vi "Periodic Tasks.vi"(8 "error in":errorcluster) -> ()   [LabVIEW 2013]
doc: "This VI runs in parallel to other tasks. It can contain as many user-defined periodic loops as you need. These can carry out PID or other sorts of timed response."
uses:
  <vilib>/Rock Robotics/WPI/DriverStation/DriverStationLCD/WPI_DriverStationLCDLCDLine.ctl
  <vilib>/Rock Robotics/SystemInterfaces/Utilities/FPGA_UtilitiesLED Source.ctl
  <vilib>/Rock Robotics/SystemInterfaces/Utilities/FPGA_UtilitiesLED State.ctl
  <vilib>/Rock Robotics/WPI/DriverStation/WPI_DriverStationRobotMode2.ctl
  <vilib>/Rock Robotics/WPI/SafetyOutput/WPI_SafetyOutputConfigMenu.ctl
  <vilib>/Rock Robotics/WPI/Solenoid/WPI_SolenoidValue.ctl
  <vilib>/Rock Robotics/WPI/Relay/WPI_RelayValue.ctl
  Begin/Global Refnums.vi
  Begin/Robot Global Data.vi
  <vilib>/Rock Robotics/WPI/Solenoid/WPI_SolenoidSetEnum.vi
  Begin/Global Variables.vi
  <vilib>/Rock Robotics/WPI/Joystick/WPI_JoystickGetSetRefNum.vi
  <vilib>/Rock Robotics/WPI/Compressor/WPI_CompressorGetSetRefNum.vi
panel:
  out "Fire":bool
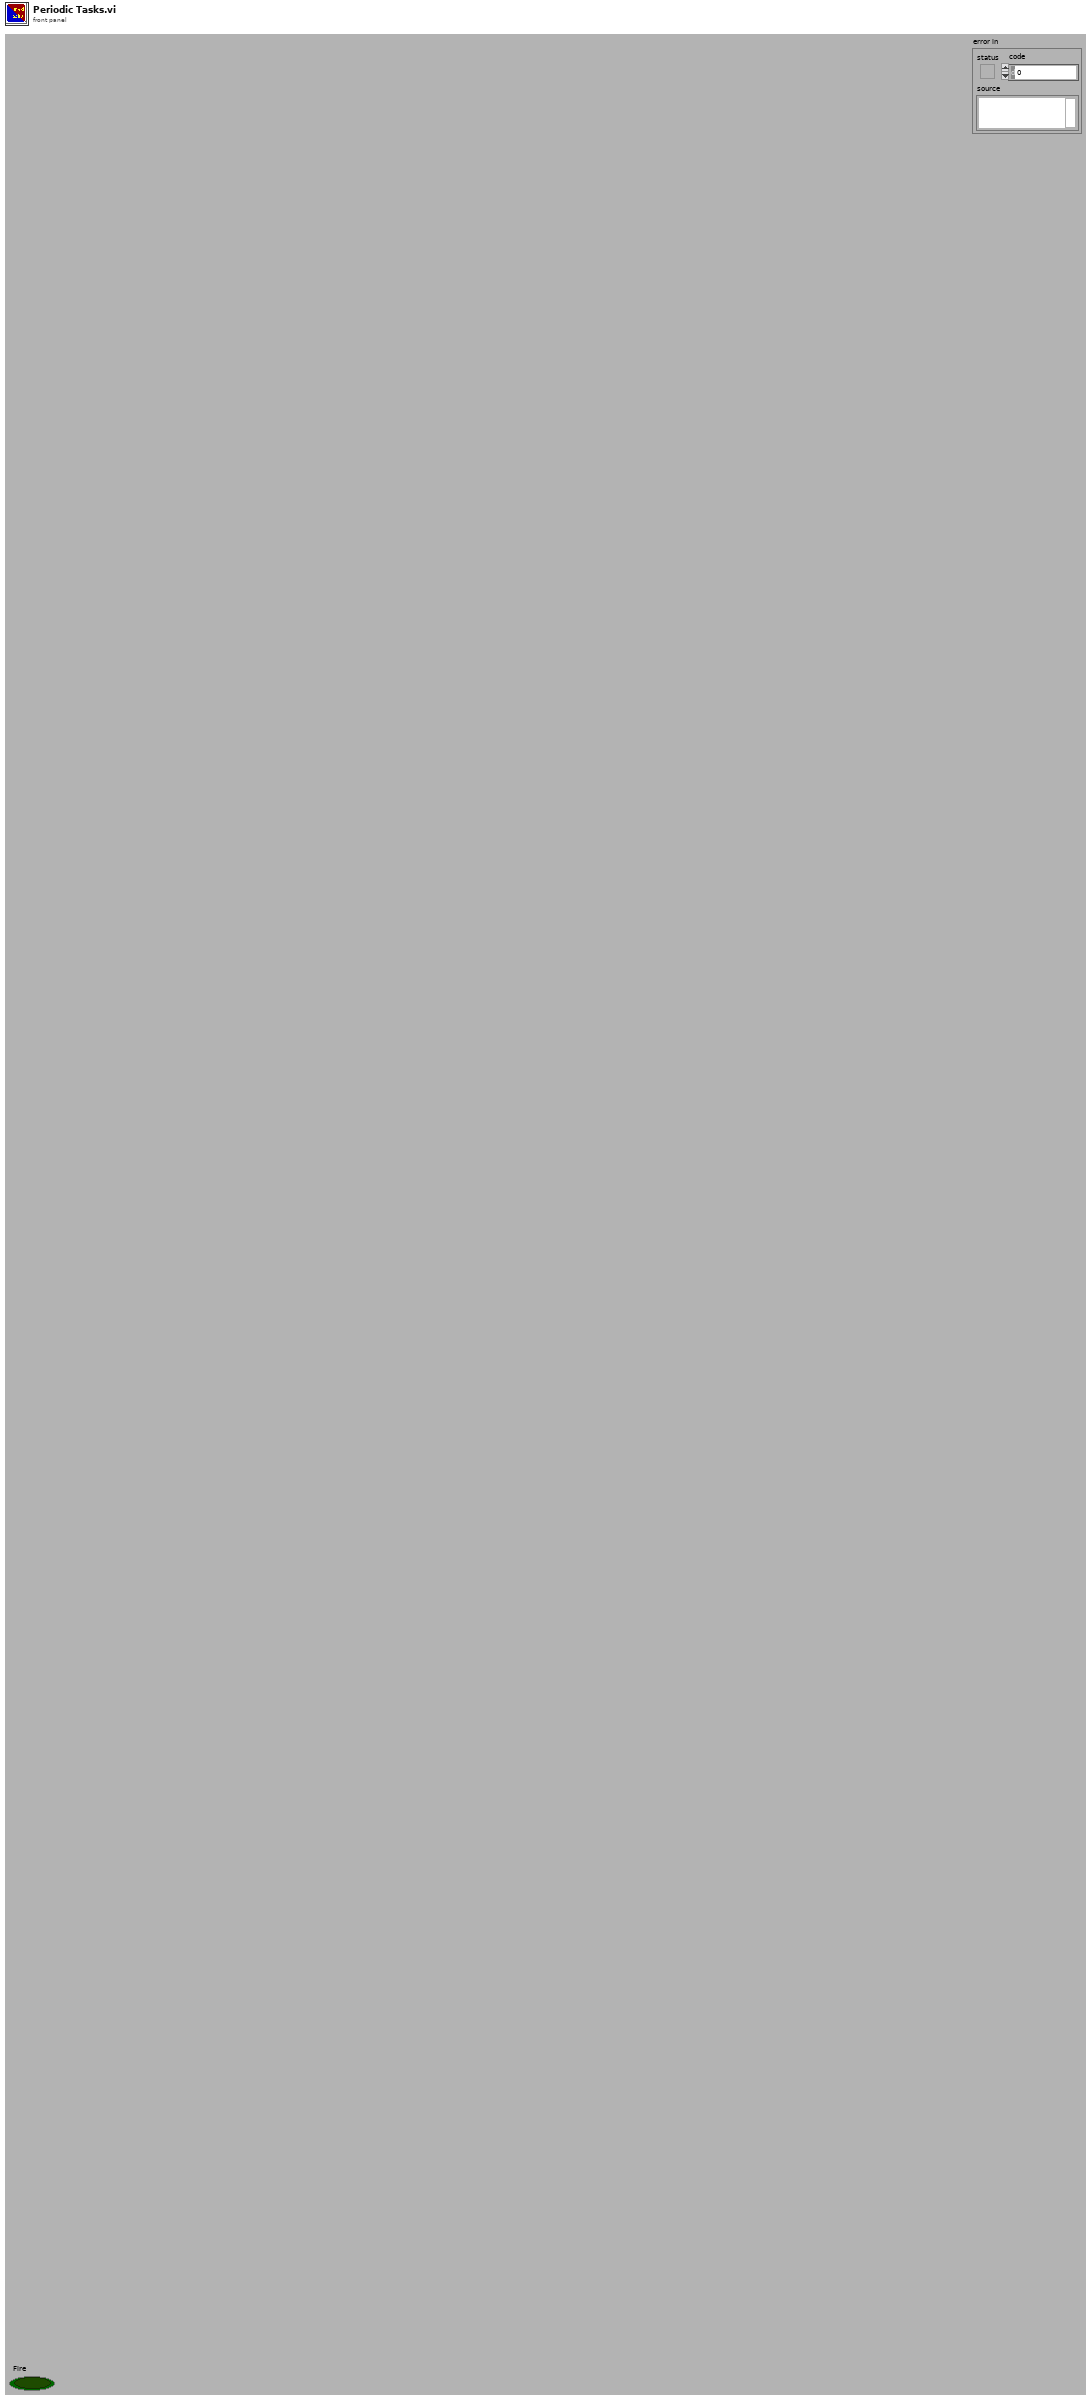
[diagram p1: front panel]
types:
  T1 = typedef "WPI_DriverStationLCDLCDLine.ctl" = enum16{"Main - Line 1", "User - Line 2", "User - Line 3", "User - Line 4", "User - Line 5", "User - Line 6"}
  T2 = typedef "WPI_DriverStationRobotMode2.ctl" = enum16{"Autonomous Disabled", "Autonomous Enabled", "Teleop Disabled", "Teleop Enabled", "Timeout", "Finish", "Test Disabled", "Test Enabled"}
  T3 = typedef "WPI_CompressorDevRef.ctl" = cluster{"DevStatus":errorcluster, "DigitalInputDevRef":T4, "RelayDevRef":T7}
  T4 = typedef "WPI_DigitalInputDevRef.ctl" = cluster{"DevStatus":errorcluster, "DIO Channel":T5, "Digital Module":T6}
  T5 = typedef "FPGA_DIOChannel.ctl" = enum8{"DIO 1", "DIO 2", "DIO 3", "DIO 4", "DIO 5", "DIO 6", "DIO 7", "DIO 8", "DIO 9", "DIO 10", "DIO 11", "DIO 12", "DIO 13", "DIO 14", "Invalid"}
  T6 = typedef "FPGA_TypedefDigitalModule.ctl" = enum16{"Digital Module 1", "Digital Module 2"}
  T7 = typedef "WPI_RelayDevRef.ctl" = cluster{"DevStatus":errorcluster, "Relay Channel":T8, "Digital Module":T6, "Relay Direction":T9}
  T8 = typedef "FPGA_DIORelayChannel.ctl" = enum8{"Relay 1", "Relay 2", "Relay 3", "Relay 4", "Relay 5", "Relay 6", "Relay 7", "Relay 8", "Invalid"}
  T9 = typedef "WPI_RelayDirection.ctl" = enum16{"Both directions", "Forward only", "Reverse only"}
  T10 = typedef "WPI_SolenoidValue.ctl" = enum16{"Off", "On", "Forward", "Reverse"}
  T11 = typedef "WPI_SafetyOutputConfigMenu.ctl" = enum16{"Enable", "Disable"}
  T12 = typedef "WPI_SolenoidDevRef.ctl" = cluster{"DevStatus":errorcluster, "Solenoid Module":T13, "Forward Solenoid Channel":T14, "Reverse Solenoid Channel":T14}
  T13 = typedef "FPGA_TypedefSolenoidModule.ctl" = enum16{"Solenoid Module 1", "Solenoid Module 2"}
  T14 = typedef "WPI_SolenoidChannel.ctl" = enum8{"Solenoid 1", "Solenoid 2", "Solenoid 3", "Solenoid 4", "Solenoid 5", "Solenoid 6", "Solenoid 7", "Solenoid 8", "Invalid"}
  T15 = typedef "WPI_RelayValue.ctl" = enum16{"Off", "On", "Forward", "Reverse"}
  T16 = typedef "WPI_EncoderDevRef.ctl" = cluster{"DevStatus":errorcluster, "EncoderIndex":T17, "CounterIndex":T18, "DistancePerCount":dbl, "Decoding Type":T19}
  T17 = typedef "FPGA_EncoderIdx.ctl" = enum8{"Enc 0", "Enc 1", "Enc 2", "Enc 3", "Invalid"}
  T18 = typedef "FPGA_CounterCtrSystemIndex.ctl" = enum8{"Ctr 0", "Ctr 1", "Ctr 2", "Ctr 3", "Ctr 4", "Ctr 5", "Ctr 6", "Ctr 7", "Invalid"}
  T19 = typedef "WPI_EncoderType.ctl" = enum16{"1x", "2x", "4x"}
  T20 = typedef "WPI_JoystickDevRef.ctl" = cluster{"Device":T21}
  T21 = typedef "WPI_JoystickDeviceEnum.ctl" = enum16{"USB 1", "USB 2", "USB 3", "USB 4", "Kinect 1", "Kinect 2"}
  T22 = typedef "WPI_JoystickButtonState.ctl" = cluster{"Button 1":bool, "Button 2":bool, "Button 3":bool, "Button 4":bool, "Button 5":bool, "Button 6":bool, "Button 7":bool, "Button 8":bool, "Button 9":bool, "Button 10":bool, "Button 11":bool, "Button 12":bool}
  T23 = typedef "WPI_MotorControlDeviceRef.ctl" = cluster{"DeviceStatus":errorcluster, "Type":enum16{"PWM", "CAN"}, "PWM":cluster{"Digital Module":T6, "PWM Channel":T24, "DeadBand":T25}, "CAN":cluster{"Device Number":u8, "Control Mode":T26, "Semaphore":T27, "Max Vout":dbl}, "Invert":bool, "TransformRef":T28, "InvTransformRef":T28}
  T24 = typedef "FPGA_DIOPWMChannel.ctl" = enum8{"PWM 1", "PWM 2", "PWM 3", "PWM 4", "PWM 5", "PWM 6", "PWM 7", "PWM 8", "PWM 9", "PWM 10", "Invalid"}
  T25 = typedef "WPI_PWMDeadband.ctl" = cluster{"Name":string, "maxPositivePwm":i32, "minPositivePwm":i32, "centerPwm":i32, "maxNegativePwm":i32, "minNegativePwm":i32, "angularRange":u16}
  T26 = typedef "WPI_CANJaguar_ControlMode.ctl" = enum8{"Percent VBus", "Current", "Speed", "Position", "Voltage"}
  T27 = typedef "Semaphore RefNum" = refnum<k1>
  T28 = typedef "WPI_PWMTransform_ConPane.ctl" = refnum<vi>
  T29 = typedef "FPGA_UtilitiesLED State.ctl" = enum16{"Off", "On", "Toggle"}
  T30 = typedef "FPGA_UtilitiesLED Source.ctl" = enum16{"User LED", "FPGA LED"}
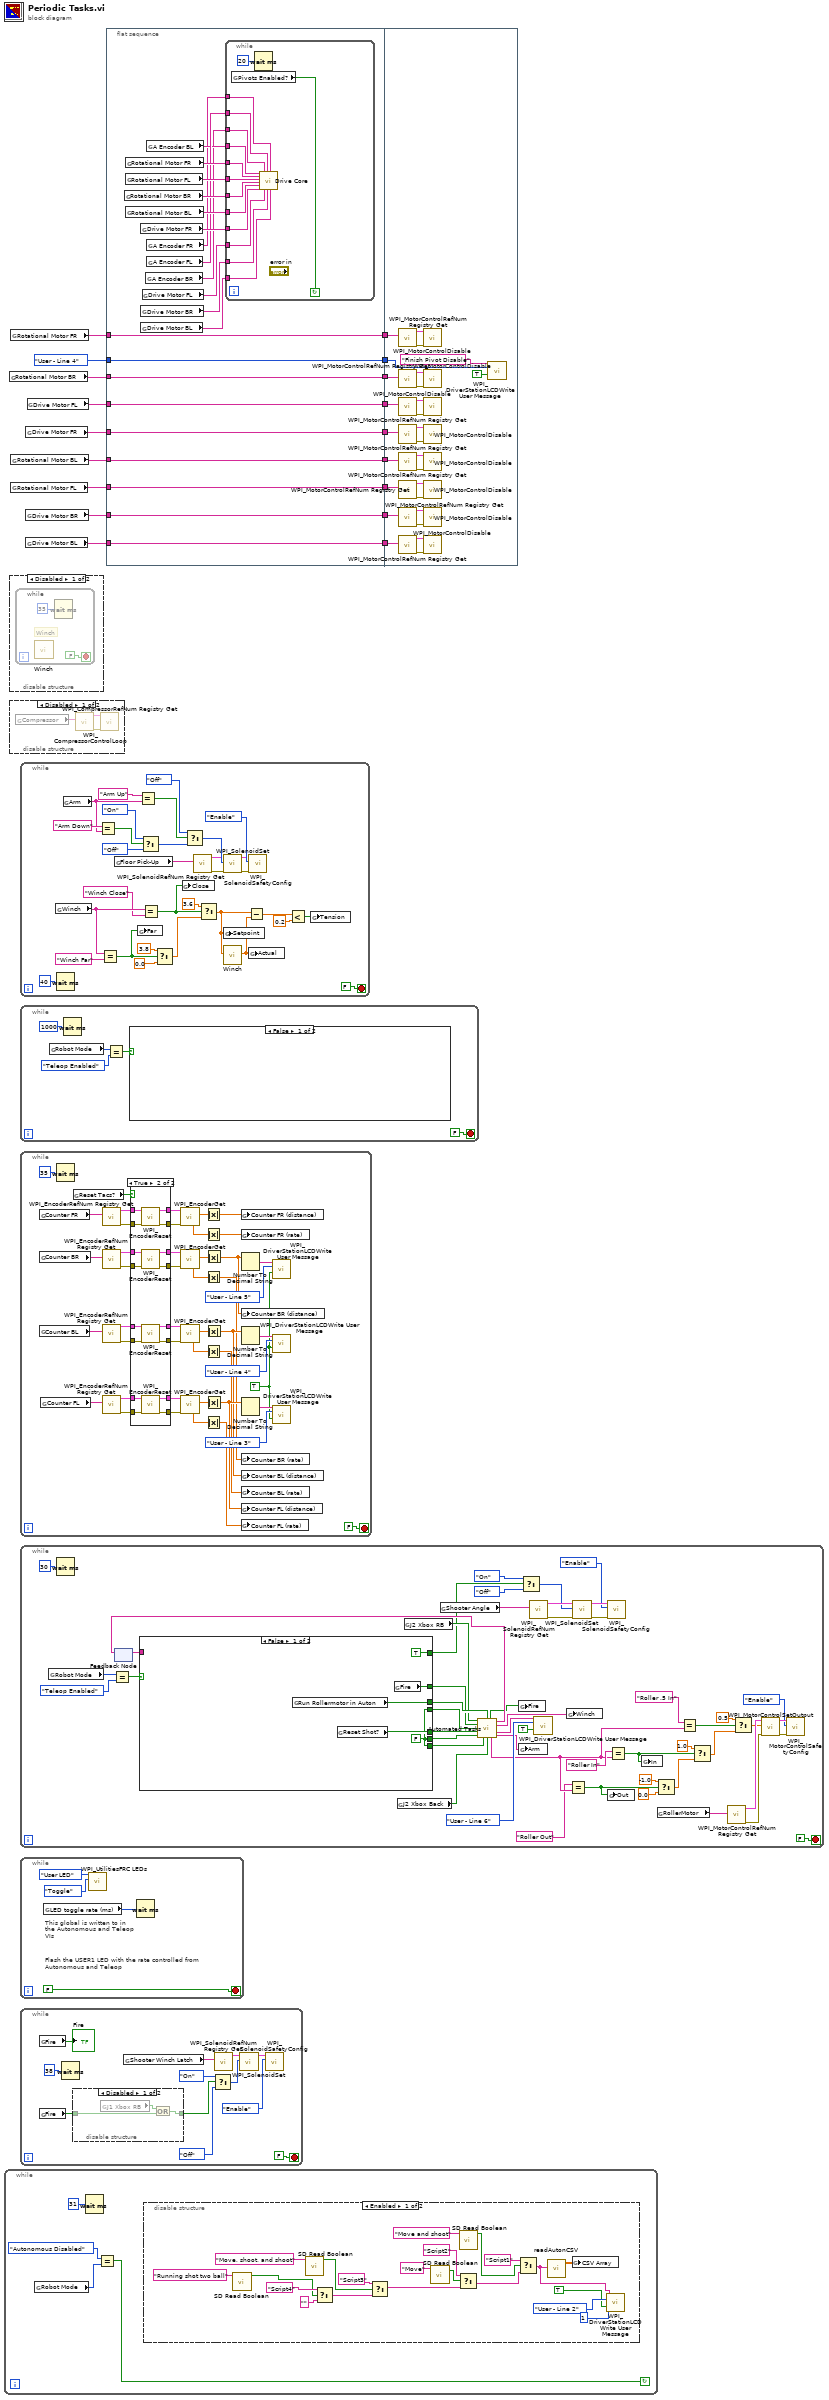
[diagram p0: block diagram]
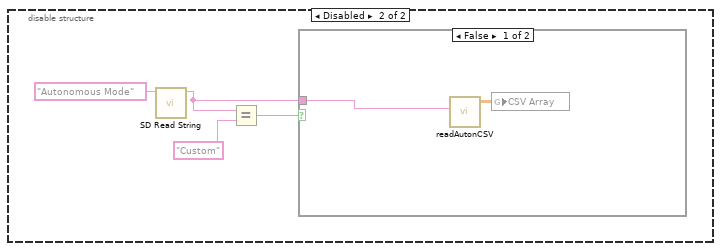
[diagram p2: hidden frame]
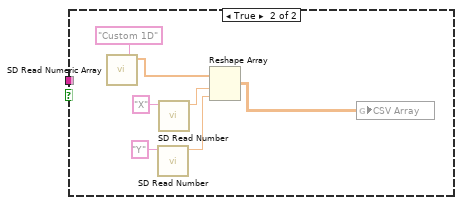
[diagram p3: hidden frame]
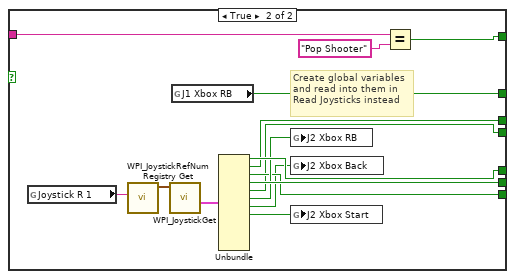
[diagram p6: hidden frame]
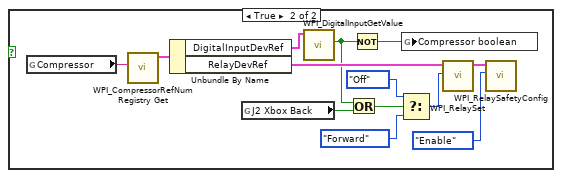
[diagram p8: hidden frame]
diagram:
  n1 = while {
    stop <- w19 continue-if-true
    n2 = global read "Robot Global Data.vi" "Robot Mode"() -> (w21:T2)
    n3 = Wait (ms)(milliseconds to wait=u32 31) -> ()  [unwired: 1 out]
    n4 = Equal?(x=WPI_DriverStationRobotMode2."Autonomous Disabled" ("y"), y=w21) -> (x = y?=w19:bool)
    n5 = disable-structure shown="Enabled" {
      frame Enabled {
        n6 = call <vilib>:"SD Read Boolean.vi"("Name"="Running shot two ball") -> ("Boolean"=w31:bool)  [unwired: 8 in, 2 out]
        n7 = call <vilib>:"SD Read Boolean.vi"("Name"="Move, shoot, and shoot") -> ("Boolean"=w36:bool)  [unwired: 8 in, 2 out]
        n8 = Select(t="Script4" ("Name"), s=w31, f="" ("Name")) -> (s? t:f=w29:string)
        n9 = Select(t="Script3" ("Name"), s=w36, f=w29) -> (s? t:f=w34:string)
        n10 = call <vilib>:"SD Read Boolean.vi"("Name"="Move") -> ("Boolean"=w41:bool)  [unwired: 8 in, 2 out]
        n11 = call <vilib>:"SD Read Boolean.vi"("Name"="Move and shoot") -> ("Boolean"=w39:bool)  [unwired: 8 in, 2 out]
        n12 = Select(t="Script2" ("Name"), s=w41, f=w34) -> (s? t:f=w40:string)
        n13 = Select(t="Script1" ("Name"), s=w39, f=w40) -> (s? t:f=w24:string)
        n14 = call "readAutonCSV.vi"("AutonFile"=w24) -> ("AutonArray"=w27:dbl[][])  [unwired: 7 in]
        n15 = global write "Global Refnums.vi" "CSV Array"(w27) -> ()
        n16 = call <vilib>:"WPI_DriverStationLCDWrite User Message.vi"("line text"=w24, "line"=WPI_DriverStationLCDLCDLine."User - Line 2", "starting column"=i8 1, "clear line before write (T)"=TRUE) -> ()  [unwired: 11 in, 1 out]
      }
      frame Disabled {
        n17 = call <vilib>:"SD Read String.vi"("Name"="Autonomous Mode") -> ("String"=w44:string)  [unwired: 8 in, 2 out]
        n18 = Equal?(x=w44, y="Custom") -> (x = y?=w45:bool)
        n19 = case shown="False" w45 {
          tunnel: w44 -> [w48 _]
          frame False {
            n20 = call "readAutonCSV.vi"("AutonFile"=w48) -> ("AutonArray"=w49:dbl[][])  [unwired: 7 in]
            n21 = global write "Global Refnums.vi" "CSV Array"(w49) -> ()
          }
          frame True {
            n22 = call <vilib>:"SD Read Numeric Array.vi"("Name"="Custom 1D") -> ("Numeric Array"=w55:dbl[])  [unwired: 8 in, 2 out]
            n23 = call <vilib>:"SD Read Number.vi"("Name"="Y") -> ("Numeric"=w51:dbl)  [unwired: 8 in, 2 out]
            n24 = call <vilib>:"SD Read Number.vi"("Name"="X") -> ("Numeric"=w54:dbl)  [unwired: 8 in, 2 out]
            n25 = Reshape Array(w55, w54, w51) -> (w50:dbl[][])
            n26 = global write "Global Refnums.vi" "CSV Array"(w50) -> ()
          }
        }
      }
    }
  }
  n27 = global read "Global Refnums.vi" "Rotational Motor BR"() -> (w16:string)
  n28 = disable-structure shown="Disabled" {
    frame Disabled {
      n29 = while {
        stop <- FALSE stop-if-true
        # "Winch"
        n30 = call "Winch.vi"() -> ()  [unwired: 11 in, 1 out]
        n31 = Wait (ms)(milliseconds to wait=u32 35) -> ()  [unwired: 1 out]
      }
    }
    frame Enabled {
    }
  }
  n32 = disable-structure shown="Disabled" {
    frame Disabled {
      n33 = global read "Global Refnums.vi" "Compressor"() -> (w61:string)
      n34 = call <vilib>:"WPI_CompressorRefNum Registry Get.vi"("refnum name"=w61) -> ("error out"=w60:errorcluster, "CompressorDevRef"=w59:T3)  [unwired: 9 in]
      n35 = call <vilib>:"WPI_CompressorControlLoop.vi"("error in (no error)"=w60, "CompressorDevRef"=w59) -> ()  [unwired: 10 in]
    }
    frame Enabled {
    }
  }
  n36 = global read "Global Refnums.vi" "Rotational Motor FR"() -> (w18:string)
  n37 = global read "Global Refnums.vi" "Rotational Motor BL"() -> (w15:string)
  n38 = global read "Global Refnums.vi" "Rotational Motor FL"() -> (w17:string)
  n39 = while {
    stop <- FALSE stop-if-true
    n40 = global read "Global Refnums.vi" "Winch"() -> (w93:string)
    n41 = Wait (ms)(milliseconds to wait=u32 40) -> ()  [unwired: 1 out]
    n42 = global read "Global Refnums.vi" "Arm"() -> (w67:string)
    n43 = Equal?(x="Arm Down", y=w67) -> (x = y?=w71:bool)
    n44 = Equal?(x=w93, y="Winch Far") -> (x = y?=w64:bool)
    n45 = global read "Global Refnums.vi" "Floor Pick-Up"() -> (w82:string)
    n46 = global write "Global Refnums.vi" "Far"(w64) -> ()
    n47 = Equal?(x="Arm Up", y=w67) -> (x = y?=w84:bool)
    n48 = Select(t=WPI_SolenoidValue."On" ("Value"), s=w71, f=WPI_SolenoidValue."Off" ("Value")) -> (s? t:f=w70:T10)
    n49 = Equal?(x=w93, y="Winch Close") -> (x = y?=w63:bool)
    n50 = Select(t=3.8, s=w64, f=0.0) -> (s? t:f=w90:dbl)
    n51 = global write "Global Refnums.vi" "Close"(w63) -> ()
    n52 = Select(t=WPI_SolenoidValue."Off" ("Value"), s=w84, f=w70) -> (s? t:f=w86:T10)
    n53 = call <vilib>:"WPI_SolenoidRefNum Registry Get.vi"("refnum name"=w82) -> ("error out"=w77:errorcluster, "SolenoidDevRef"=w78:T12)  [unwired: 9 in]
    n54 = Select(t=3.6, s=w63, f=w90) -> (s? t:f=w62:dbl)
    n55 = call-poly <vilib>:"WPI_SolenoidSet.vi"("error in (no error)"=w77, "Value"=w86, "SolenoidDevRef"=w78) -> ("error out"=w80:errorcluster, "SolenoidDevRef"=w79:T12)  [unwired: 7 in]
    n56 = global write "Global Refnums.vi" "Setpoint"(w62) -> ()
    n57 = call "Winch.vi"("setpoint"=w62) -> ("Actual"=w65:dbl)  [unwired: 10 in]
    n58 = Subtract(x=w62, y=w65) -> (x-y=w74:dbl)
    n59 = call <vilib>:"WPI_SolenoidSafetyConfig.vi"("error in (no error)"=w80, "mode"=WPI_SafetyOutputConfigMenu."Enable", "SolenoidDevRef"=w79) -> ()  [unwired: 7 in, 2 out]
    n60 = global write "Global Refnums.vi" "Actual"(w65) -> ()
    n61 = Less?(x=w74, y=0.2) -> (x < y?=w66:bool)
    n62 = global write "Global Refnums.vi" "Tension"(w66) -> ()
  }
  n63 = while {
    stop <- FALSE stop-if-true
    n64 = global read "Robot Global Data.vi" "Robot Mode"() -> (w96:T2)
    n65 = Wait (ms)(milliseconds to wait=1000) -> ()  [unwired: 1 out]
    n66 = Equal?(x=w96, y=WPI_DriverStationRobotMode2."Teleop Enabled") -> (x = y?=w94:bool)
    n67 = case shown="False" w94 {
      frame False {
      }
      frame True {
        n68 = global read "Global Refnums.vi" "Compressor"() -> (w111:string)
        n69 = call <vilib>:"WPI_CompressorRefNum Registry Get.vi"("refnum name"=w111) -> ("CompressorDevRef"=w110:T3)  [unwired: 9 in, 1 out]
        n70 = Unbundle By Name(w110) -> ("DigitalInputDevRef"=w103:T4, "RelayDevRef"=w109:T7)
        n71 = global read "Global Variables.vi" "J2 Xbox Back"() -> (w101:bool)
        n72 = call <vilib>:"WPI_DigitalInputGetValue.vi"("DigitalInputDevRef"=w103) -> ("Value"=w100:bool)  [unwired: 8 in, 2 out]
        n73 = Or(x=w100, y=w101) -> (x .or. y?=w102:bool)
        n74 = Not(x=w100) -> (.not. x?=w99:bool)
        n75 = Select(t=WPI_RelayValue."Off" ("RelayValue"), s=w102, f=WPI_RelayValue."Forward" ("RelayValue")) -> (s? t:f=w106:T15)
        n76 = global write "Global Refnums.vi" "Compressor boolean"(w99) -> ()
        n77 = call <vilib>:"WPI_RelaySet.vi"("RelayValue"=w106, "RelayDevRef"=w109) -> ("RelayDevRef"=w108:T7)  [unwired: 8 in, 1 out]
        n78 = call <vilib>:"WPI_RelaySafetyConfig.vi"("mode"=WPI_SafetyOutputConfigMenu."Enable", "RelayDevRef"=w108) -> ()  [unwired: 8 in, 2 out]
      }
    }
  }
  n79 = while {
    stop <- FALSE stop-if-true
    w113 = TRUE ("clear line before write (T)")
    n80 = global read "Global Refnums.vi" "Counter FR"() -> (w124:string)
    n81 = global read "Global Refnums.vi" "Counter BR"() -> (w122:string)
    n82 = global read "Global Refnums.vi" "Counter BL"() -> (w125:string)
    n83 = global read "Global Refnums.vi" "Counter FL"() -> (w123:string)
    n84 = Wait (ms)(milliseconds to wait=u32 35) -> ()  [unwired: 1 out]
    n85 = global read "Global Variables.vi" "Reset Tacs?"() -> (w112:bool)
    n86 = call <vilib>:"WPI_EncoderRefNum Registry Get.vi"("refnum name"=w124) -> ("error out"=w140:errorcluster, "EncoderDevRef"=w143:T16)  [unwired: 9 in]
    n87 = call <vilib>:"WPI_EncoderRefNum Registry Get.vi"("refnum name"=w122) -> ("error out"=w148:errorcluster, "EncoderDevRef"=w149:T16)  [unwired: 9 in]
    n88 = call <vilib>:"WPI_EncoderRefNum Registry Get.vi"("refnum name"=w125) -> ("error out"=w150:errorcluster, "EncoderDevRef"=w151:T16)  [unwired: 9 in]
    n89 = call <vilib>:"WPI_EncoderRefNum Registry Get.vi"("refnum name"=w123) -> ("error out"=w145:errorcluster, "EncoderDevRef"=w146:T16)  [unwired: 9 in]
    n90 = case shown="True" w112 {
      tunnel: w149 -> [w162 w181]
      tunnel: [w162 w180] -> w154
      tunnel: [w164 w179] -> w155
      tunnel: w148 -> [w164 w178]
      tunnel: [w163 w177] -> w153
      tunnel: [w165 w176] -> w152
      tunnel: w151 -> [w163 w175]
      tunnel: w150 -> [w165 w174]
      tunnel: [w161 w166] -> w147
      tunnel: w146 -> [w161 w173]
      tunnel: w145 -> [w160 w172]
      tunnel: [w160 w167] -> w144
      tunnel: w143 -> [w159 w171]
      tunnel: [w159 w168] -> w142
      tunnel: [w158 w169] -> w141
      tunnel: w140 -> [w158 w170]
      frame False {
      }
      frame True {
        n91 = call <vilib>:"WPI_EncoderReset.vi"("error in (no error)"=w170, "EncoderDevRef"=w171) -> ("error out"=w169:errorcluster, "EncoderDevRef"=w168:T16)  [unwired: 8 in]
        n92 = call <vilib>:"WPI_EncoderReset.vi"("error in (no error)"=w178, "EncoderDevRef"=w181) -> ("error out"=w179:errorcluster, "EncoderDevRef"=w180:T16)  [unwired: 8 in]
        n93 = call <vilib>:"WPI_EncoderReset.vi"("error in (no error)"=w174, "EncoderDevRef"=w175) -> ("error out"=w176:errorcluster, "EncoderDevRef"=w177:T16)  [unwired: 8 in]
        n94 = call <vilib>:"WPI_EncoderReset.vi"("error in (no error)"=w172, "EncoderDevRef"=w173) -> ("error out"=w167:errorcluster, "EncoderDevRef"=w166:T16)  [unwired: 8 in]
      }
    }
    n95 = call <vilib>:"WPI_EncoderGet.vi"("error in (no error)"=w141, "EncoderDevRef"=w142) -> ("Distance"=w137:dbl, "Rate"=w133:dbl)  [unwired: 4 in, 4 out]
    n96 = call <vilib>:"WPI_EncoderGet.vi"("error in (no error)"=w155, "EncoderDevRef"=w154) -> ("Distance"=w136:dbl, "Rate"=w132:dbl)  [unwired: 4 in, 4 out]
    n97 = call <vilib>:"WPI_EncoderGet.vi"("error in (no error)"=w152, "EncoderDevRef"=w153) -> ("Distance"=w138:dbl, "Rate"=w134:dbl)  [unwired: 4 in, 4 out]
    n98 = call <vilib>:"WPI_EncoderGet.vi"("error in (no error)"=w144, "EncoderDevRef"=w147) -> ("Distance"=w139:dbl, "Rate"=w135:dbl)  [unwired: 4 in, 4 out]
    n99 = Absolute Value(x=w137) -> (abs(x)=w121:dbl)
    n100 = Absolute Value(x=w133) -> (abs(x)=w120:dbl)
    n101 = Absolute Value(x=w132) -> (abs(x)=w114:dbl)
    n102 = Absolute Value(x=w134) -> (abs(x)=w116:dbl)
    n103 = Absolute Value(x=w135) -> (abs(x)=w118:dbl)
    n104 = Absolute Value(x=w136) -> (abs(x)=w115:dbl)
    n105 = Absolute Value(x=w138) -> (abs(x)=w117:dbl)
    n106 = Absolute Value(x=w139) -> (abs(x)=w119:dbl)
    n107 = global write "Global Refnums.vi" "Counter FR (distance)"(w121) -> ()
    n108 = global write "Global Refnums.vi" "Counter FR (rate)"(w120) -> ()
    n109 = Number To Decimal String(number=w115) -> (decimal integer string=w131:string)  [unwired: 1 in]
    n110 = global write "Global Refnums.vi" "Counter BR (distance)"(w115) -> ()
    n111 = Number To Decimal String(number=w117) -> (decimal integer string=w129:string)  [unwired: 1 in]
    n112 = Number To Decimal String(number=w119) -> (decimal integer string=w130:string)  [unwired: 1 in]
    n113 = global write "Global Refnums.vi" "Counter BR (rate)"(w114) -> ()
    n114 = global write "Global Refnums.vi" "Counter BL (distance)"(w117) -> ()
    n115 = global write "Global Refnums.vi" "Counter BL (rate)"(w116) -> ()
    n116 = global write "Global Refnums.vi" "Counter FL (distance)"(w119) -> ()
    n117 = global write "Global Refnums.vi" "Counter FL (rate)"(w118) -> ()
    n118 = call <vilib>:"WPI_DriverStationLCDWrite User Message.vi"("line text"=w131, "line"=WPI_DriverStationLCDLCDLine."User - Line 5", "clear line before write (T)"=w113) -> ()  [unwired: 12 in, 1 out]
    n119 = call <vilib>:"WPI_DriverStationLCDWrite User Message.vi"("line text"=w129, "line"=WPI_DriverStationLCDLCDLine."User - Line 4", "clear line before write (T)"=w113) -> ()  [unwired: 12 in, 1 out]
    n120 = call <vilib>:"WPI_DriverStationLCDWrite User Message.vi"("line text"=w130, "line"=WPI_DriverStationLCDLCDLine."User - Line 3", "clear line before write (T)"=w113) -> ()  [unwired: 12 in, 1 out]
  }
  n121 = while {
    stop <- FALSE stop-if-true
    n122 = global read "Robot Global Data.vi" "Robot Mode"() -> (w203:T2)
    n123 = Wait (ms)(milliseconds to wait=u32 30) -> ()  [unwired: 1 out]
    n124 = Equal?(x=w203, y=WPI_DriverStationRobotMode2."Teleop Enabled") -> (x = y?=w204:bool)
    n125 = feedback #1() -> (w199:string)  [unwired: 1 in]
    n126 = case shown="False" w204 {
      tunnel: [w234 w249] -> w187
      tunnel: [w236 w248] -> w215
      tunnel: [w233 w247] -> w214
      tunnel: [w237 w246] -> w213
      tunnel: w199 -> [_ w244]
      tunnel: [TRUE w243] -> w198
      tunnel: [w233 w241] -> w196
      tunnel: [w233 w240] -> w188
      frame False {
        w233 = FALSE ("J1 Xbox RB")
        n127 = global read "Global Refnums.vi" "Run Rollermotor in Auton"() -> (w236:bool)
        n128 = global read "Global Refnums.vi" "Reset Shot?"() -> (w234:bool)
        n129 = global read "Global Refnums.vi" "Fire"() -> (w237:bool)
      }
      frame True {
        # "Create global variables\nand read into them in \nRead Joysticks instead"
        n130 = global read "Global Refnums.vi" "Joystick R 1"() -> (w250:string)
        n131 = call <vilib>:"WPI_JoystickRefNum Registry Get.vi"("refnum name"=w250) -> ("JoystickDevRef"=w252:T20)  [unwired: 9 in, 1 out]
        n132 = call <vilib>:"WPI_JoystickGet.vi"("JoystickDevRef"=w252) -> ("Buttons"=w251:T22)  [unwired: 4 in, 2 out]
        n133 = global read "Global Variables.vi" "J1 Xbox RB"() -> (w246:bool)
        n134 = Unbundle(w251) -> ("Button 1"=w249:bool, "Button 2"=w248:bool, "Button 3"=w241:bool, "Button 4"=w247:bool, "Button 5"=w240:bool, "Button 6"=w242:bool, "Button 7"=w239:bool, "Button 8"=w238:bool)  [unwired: 4 out]
        n135 = global write "Global Variables.vi" "J2 Xbox RB"(w242) -> ()
        n136 = global write "Global Variables.vi" "J2 Xbox Back"(w239) -> ()
        n137 = global write "Global Variables.vi" "J2 Xbox Start"(w238) -> ()
        n138 = Equal?(x=w244, y="Pop Shooter") -> (x = y?=w243:bool)
      }
    }
    n139 = global read "Global Variables.vi" "J2 Xbox Back"() -> (w184:bool)
    n140 = global read "Global Variables.vi" "J2 Xbox RB"() -> (w201:bool)
    n141 = global read "Global Refnums.vi" "Shooter Angle"() -> (w211:string)
    n142 = call "Automated Tasks.vi"("RB"=w201, "B"=w215, "Fire"=w213, "LB"=w188, "A"=w187, "Y"=w214, "X"=w196, "Back"=w184) -> ("Fire"=w197:bool, "Shooter"=w200:string, "Winch"=w186:string, "Case"=w209:string, "Roller"=w193:string, "Arm"=w206:string)  [unwired: 2 in]
    n143 = feedback-in #1(w200) -> ()
    n144 = global write "Global Refnums.vi" "Fire"(w197) -> ()
    n145 = global write "Global Refnums.vi" "Arm"(w206) -> ()
    n146 = Select(t=WPI_SolenoidValue."On" ("Value"), s=w198, f=WPI_SolenoidValue."Off" ("Value")) -> (s? t:f=w216:T10)
    n147 = call <vilib>:"WPI_SolenoidRefNum Registry Get.vi"("refnum name"=w211) -> ("error out"=w223:errorcluster, "SolenoidDevRef"=w222:T12)  [unwired: 9 in]
    n148 = call <vilib>:"WPI_DriverStationLCDWrite User Message.vi"("line text"=w209, "line"=WPI_DriverStationLCDLCDLine."User - Line 6", "clear line before write (T)"=TRUE) -> ()  [unwired: 12 in, 1 out]
    n149 = global write "Global Refnums.vi" "Winch"(w186) -> ()
    n150 = Equal?(x="Roller Out", y=w193) -> (x = y?=w182:bool)
    n151 = call-poly <vilib>:"WPI_SolenoidSet.vi"("error in (no error)"=w223, "Value"=w216, "SolenoidDevRef"=w222) -> ("error out"=w220:errorcluster, "SolenoidDevRef"=w221:T12)  [unwired: 7 in]
    n152 = call <vilib>:"WPI_SolenoidSafetyConfig.vi"("error in (no error)"=w220, "mode"=WPI_SafetyOutputConfigMenu."Enable", "SolenoidDevRef"=w221) -> ()  [unwired: 7 in, 2 out]
    n153 = global write "Global Refnums.vi" "Out"(w182) -> ()
    n154 = Equal?(x="Roller In", y=w193) -> (x = y?=w183:bool)
    n155 = global write "Global Refnums.vi" "In"(w183) -> ()
    n156 = Select(t=-1.0, s=w182, f=0.0) -> (s? t:f=w224:dbl)
    n157 = global read "Global Refnums.vi" "RollerMotor"() -> (w212:string)
    n158 = Equal?(x="Roller .5 In", y=w193) -> (x = y?=w192:bool)
    n159 = Select(t=1.0, s=w183, f=w224) -> (s? t:f=w191:dbl)
    n160 = call <vilib>:"WPI_MotorControlRefNum Registry Get.vi"("refnum name"=w212) -> ("error out"=w230:errorcluster, "MotorControlDevRef"=w232:T23)  [unwired: 9 in]
    n161 = Select(t=0.5, s=w192, f=w191) -> (s? t:f=w195:dbl)
    n162 = call <vilib>:"WPI_MotorControlSetOutput.vi"("error in (no error)"=w230, "Output"=w195, "MotorControlDevRef"=w232) -> ("error out"=w229:errorcluster, "MotorControlDevRef"=w231:T23)  [unwired: 6 in, 1 out]
    n163 = call <vilib>:"WPI_MotorControlSafetyConfig.vi"("error in (no error)"=w229, "mode"=WPI_SafetyOutputConfigMenu."Enable", "MotorControlDevRef"=w231) -> ()  [unwired: 7 in, 2 out]
  }
  n164 = while {
    stop <- FALSE stop-if-true
    # "This global is written to in the Autonomous and Teleop VIs"
    # "Flash the USER1 LED with the rate controlled from Autonomous and Teleop"
    n165 = global read "Robot Global Data.vi" "LED toggle rate (ms)"() -> (w253:u32)
    n166 = call <vilib>:"WPI_UtilitiesFRC LEDs.vi"("State"=FPGA_UtilitiesLED_State."Toggle", "LED Type"=FPGA_UtilitiesLED_Source."User LED") -> ()  [unwired: 1 in, 9 out]
    n167 = Wait (ms)(milliseconds to wait=w253) -> ()  [unwired: 1 out]
  }
  n168 = while {
    stop <- FALSE stop-if-true
    n169 = global read "Global Refnums.vi" "Fire"() -> (→"Fire":bool)
    n170 = global read "Global Refnums.vi" "Fire"() -> (w258:bool)
    n171 = Wait (ms)(milliseconds to wait=u32 38) -> ()  [unwired: 1 out]
    n172 = disable-structure shown="Disabled" {
      disable-tunnel: w258 -> [w271 w272]
      disable-tunnel: [w269 w272] -> w257
      frame Disabled {
        n173 = global read "Global Variables.vi" "J1 Xbox RB"() -> (w270:bool)
        n174 = Or(x=w270, y=w271) -> (x .or. y?=w269:bool)
      }
      frame Enabled {
      }
    }
    n175 = global read "Global Refnums.vi" "Shooter Winch Latch"() -> (w264:string)
    n176 = Select(t=WPI_SolenoidValue."On", s=w257, f=WPI_SolenoidValue."Off" ("Value")) -> (s? t:f=w259:T10)
    n177 = call <vilib>:"WPI_SolenoidRefNum Registry Get.vi"("refnum name"=w264) -> ("SolenoidDevRef"=w265:T12)  [unwired: 9 in, 1 out]
    n178 = call-poly <vilib>:"WPI_SolenoidSet.vi"("Value"=w259, "SolenoidDevRef"=w265) -> ("SolenoidDevRef"=w266:T12)  [unwired: 8 in, 1 out]
    n179 = call <vilib>:"WPI_SolenoidSafetyConfig.vi"("mode"=WPI_SafetyOutputConfigMenu."Enable", "SolenoidDevRef"=w266) -> ()  [unwired: 8 in, 2 out]
  }
  n180 = global read "Global Refnums.vi" "Drive Motor FR"() -> (w14:string)
  n181 = global read "Global Refnums.vi" "Drive Motor BR"() -> (w12:string)
  n182 = global read "Global Refnums.vi" "Drive Motor BL"() -> (w11:string)
  n183 = global read "Global Refnums.vi" "Drive Motor FL"() -> (w13:string)
  n184 = flat-sequence {
    tunnel: WPI_DriverStationLCDLCDLine."User - Line 4" ("line") -> [w285]
    tunnel: w13 -> [w286]
    tunnel: w11 -> [w287]
    tunnel: w12 -> [w288]
    tunnel: w14 -> [w289]
    tunnel: w15 -> [w290]
    tunnel: w16 -> [w291]
    tunnel: w17 -> [w292]
    tunnel: w18 -> [w293]
    tunnel: [w293] -> w9
    tunnel: [w292] -> w8
    tunnel: [w291] -> w7
    tunnel: [w290] -> w6
    tunnel: [w289] -> w5
    tunnel: [w288] -> w4
    tunnel: [w287] -> w3
    tunnel: [w286] -> w2
    tunnel: [w285] -> w1
    tunnel: w9 -> [w334]
    tunnel: w8 -> [w327]
    tunnel: w7 -> [w326]
    tunnel: w6 -> [w323]
    tunnel: w5 -> [w314]
    tunnel: w4 -> [w313]
    tunnel: w3 -> [w312]
    tunnel: w2 -> [w311]
    tunnel: w1 -> [w310]
    frame #0 {
      n185 = global read "Global Refnums.vi" "Rotational Motor BR"() -> (w279:string)
      n186 = global read "Global Refnums.vi" "Rotational Motor FR"() -> (w277:string)
      n187 = global read "Global Refnums.vi" "Rotational Motor FL"() -> (w278:string)
      n188 = global read "Global Refnums.vi" "Rotational Motor BL"() -> (w280:string)
      n189 = global read "Global Refnums.vi" "Drive Motor FR"() -> (w281:string)
      n190 = global read "Global Refnums.vi" "Drive Motor BR"() -> (w283:string)
      n191 = global read "Global Refnums.vi" "Drive Motor BL"() -> (w284:string)
      n192 = global read "Global Refnums.vi" "Drive Motor FL"() -> (w282:string)
      n193 = global read "Global Refnums.vi" "A Encoder BR"() -> (w274:string)
      n194 = global read "Global Refnums.vi" "A Encoder BL"() -> (w275:string)
      n195 = global read "Global Refnums.vi" "A Encoder FR"() -> (w273:string)
      n196 = global read "Global Refnums.vi" "A Encoder FL"() -> (w276:string)
      n197 = while {
        tunnel: w273 -> [w307]
        tunnel: w274 -> [w305]
        tunnel: w275 -> [w304]
        tunnel: w276 -> [w306]
        tunnel: w281 -> [w299]
        tunnel: w283 -> [w297]
        tunnel: w284 -> [w296]
        tunnel: w282 -> [w298]
        tunnel: w277 -> [w303]
        tunnel: w279 -> [w301]
        tunnel: w280 -> [w300]
        tunnel: w278 -> [w302]
        stop <- w294 continue-if-true
        n198 = global read "Global Variables.vi" "Pivots Enabled?"() -> (w294:bool)
        n199 = Wait (ms)(milliseconds to wait=u32 20) -> ()  [unwired: 1 out]
        n200 = call "Drive Core.vi"("A Encoder BL"=w304, "Rotational Motor FR"=w303, "Rotational Motor FL"=w302, "Rotational Motor BR"=w301, "Rotational Motor BL"=w300, "Drive Motor FR"=w299, "A Encoder BR"=w305, "Drive Motor FL"=w298, "A Encoder FL"=w306, "Drive Motor BR"=w297, "A Encoder FR"=w307, "Drive Motor BL"=w296) -> ()  [unwired: 8 in]
      }
    }
    frame #1 {
      n201 = call <vilib>:"WPI_MotorControlRefNum Registry Get.vi"("refnum name"=w334) -> ("error out"=w332:errorcluster, "MotorControlDevRef"=w333:T23)  [unwired: 9 in]
      n202 = call <vilib>:"WPI_MotorControlRefNum Registry Get.vi"("refnum name"=w326) -> ("error out"=w328:errorcluster, "MotorControlDevRef"=w329:T23)  [unwired: 9 in]
      n203 = call <vilib>:"WPI_MotorControlRefNum Registry Get.vi"("refnum name"=w311) -> ("error out"=w318:errorcluster, "MotorControlDevRef"=w317:T23)  [unwired: 9 in]
      n204 = call <vilib>:"WPI_MotorControlRefNum Registry Get.vi"("refnum name"=w314) -> ("error out"=w316:errorcluster, "MotorControlDevRef"=w315:T23)  [unwired: 9 in]
      n205 = call <vilib>:"WPI_MotorControlRefNum Registry Get.vi"("refnum name"=w323) -> ("error out"=w324:errorcluster, "MotorControlDevRef"=w325:T23)  [unwired: 9 in]
      n206 = call <vilib>:"WPI_MotorControlRefNum Registry Get.vi"("refnum name"=w327) -> ("error out"=w330:errorcluster, "MotorControlDevRef"=w331:T23)  [unwired: 9 in]
      n207 = call <vilib>:"WPI_MotorControlRefNum Registry Get.vi"("refnum name"=w313) -> ("error out"=w320:errorcluster, "MotorControlDevRef"=w319:T23)  [unwired: 9 in]
      n208 = call <vilib>:"WPI_MotorControlRefNum Registry Get.vi"("refnum name"=w312) -> ("error out"=w322:errorcluster, "MotorControlDevRef"=w321:T23)  [unwired: 9 in]
      n209 = call <vilib>:"WPI_MotorControlDisable.vi"("error in (no error)"=w332, "MotorControlDevRef"=w333) -> ()  [unwired: 8 in, 2 out]
      n210 = call <vilib>:"WPI_MotorControlDisable.vi"("error in (no error)"=w328, "MotorControlDevRef"=w329) -> ()  [unwired: 8 in, 2 out]
      n211 = call <vilib>:"WPI_MotorControlDisable.vi"("error in (no error)"=w318, "MotorControlDevRef"=w317) -> ()  [unwired: 8 in, 2 out]
      n212 = call <vilib>:"WPI_MotorControlDisable.vi"("error in (no error)"=w316, "MotorControlDevRef"=w315) -> ()  [unwired: 8 in, 2 out]
      n213 = call <vilib>:"WPI_MotorControlDisable.vi"("error in (no error)"=w324, "MotorControlDevRef"=w325) -> ()  [unwired: 8 in, 2 out]
      n214 = call <vilib>:"WPI_MotorControlDisable.vi"("error in (no error)"=w330, "MotorControlDevRef"=w331) -> ()  [unwired: 8 in, 2 out]
      n215 = call <vilib>:"WPI_MotorControlDisable.vi"("error in (no error)"=w320, "MotorControlDevRef"=w319) -> ()  [unwired: 8 in, 2 out]
      n216 = call <vilib>:"WPI_MotorControlDisable.vi"("error in (no error)"=w322, "MotorControlDevRef"=w321) -> ()  [unwired: 8 in, 2 out]
      n217 = call <vilib>:"WPI_DriverStationLCDWrite User Message.vi"("line text"="Finish Pivot Disable", "line"=w310, "clear line before write (T)"=TRUE) -> ()  [unwired: 12 in, 1 out]
    }
  }
